vi "Fetch git abbreviated hash.vi"(8 "error in (no error)":errorcluster, 10 "git repo path":path=path "C:/", 11 "git.exe path":path=path "C:/Program Files/Git/cmd/git.exe") -> (0 "error out":errorcluster, 1 "Fetch error?":bool, 2 "Abbreviated hash":string, 3 "Output string":string)   [LabVIEW 2016]
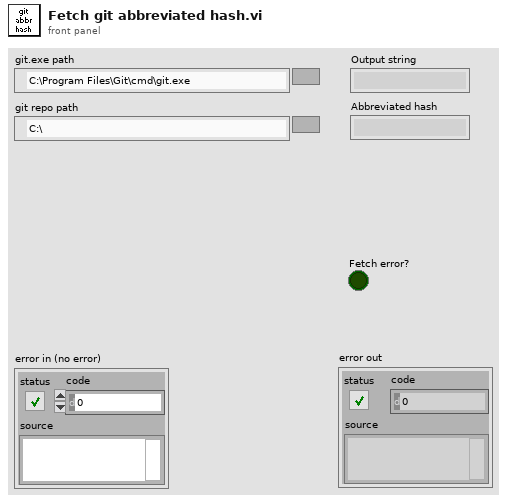
[diagram p1: front panel]
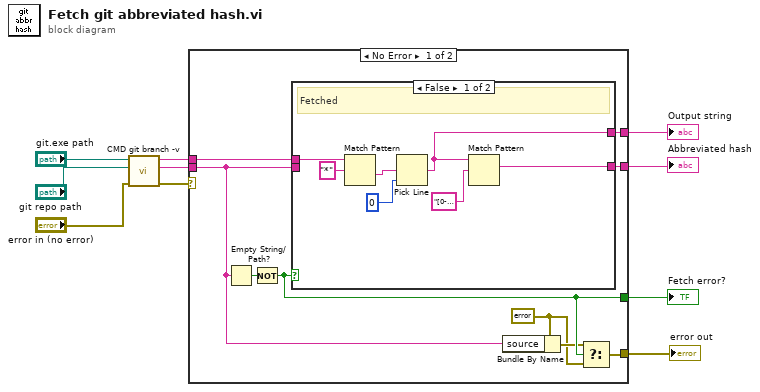
[diagram p0: block diagram]
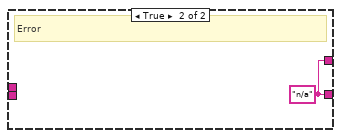
[diagram p2: hidden frame]
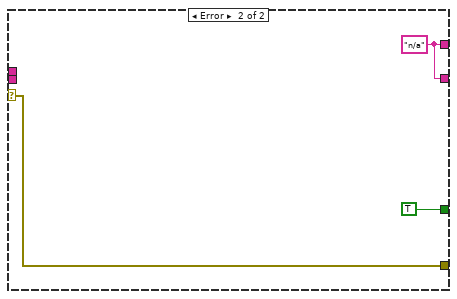
[diagram p3: hidden frame]
diagram:
  n1 = call "CMD git branch -v.vi"("error in (no error)"="error in (no error)", "git repo path"="git repo path", "git.exe path"="git.exe path") -> ("error out"=w2:errorcluster, "standard error"=w3:string, "standard output"=w4:string)  [unwired: 5 in, 1 out]
  n2 = case shown="No Error" w2 {
    selector: w2 -> [_ w29]
    tunnel: [w19 w29] -> w7
    tunnel: [w18 TRUE] -> w6
    tunnel: [w11 w28] -> w1
    tunnel: [w17 w28] -> w5
    tunnel: w4 -> [w15 _]
    tunnel: w3 -> [w13 _]
    frame No Error {
      w12 = errorcluster {"status"=FALSE, "code"=0, "source"=""} ("error in (no error)")
      n3 = Empty String/Path?(string/path=w13) -> (empty?=w16:bool)
      n4 = Not(x=w16) -> (.not. x?=w18:bool)
      n5 = case shown="False" w18 {
        tunnel: w15 -> [w26 _]
        tunnel: w13 -> [_ _]
        tunnel: [w21 w27] -> w11
        tunnel: [w20 w27] -> w17
        frame False {
          # "Fetched"
          n6 = Match Pattern(string=w26, regular expression="*") -> (after substring=w24:string)  [unwired: 1 in, 3 out]
          n7 = Pick Line(multi-line string=w24, line index=0) -> (output string=w20:string)  [unwired: 1 in]
          n8 = Match Pattern(string=w20, regular expression="[0-9abced][0-9abced][0-9abced][0-9abced][0-9abced][0-9abced][0-9abced]") -> (match substring=w21:string)  [unwired: 1 in, 3 out]
        }
        frame True {
          w27 = "n/a" ("output string")
          # "Error"
        }
      }
      n9 = Bundle By Name(cluster=w12, "source"=w13) -> (w14:errorcluster)
      n10 = Select(t=w14, s=w18, f=w12) -> (s? t:f=w19:errorcluster)
    }
    frame Error {
      w28 = "n/a" ("standard output")
    }
  }
  "Fetch error?" <- w6
  "error out" <- w7
  "Abbreviated hash" <- w1
  "Output string" <- w5
